vi "Rotate Points.vi"(0 "Points In":cluster{i32, i32}[](array[cluster]), 5 "direction":cluster{"x":i16, "y":i16}, 11 "angle":dbl) -> (4 "Rotated Points":cluster{i32, i32}[](array[cluster]))   [LabVIEW 2020, in "FSM.EdgeEnd.lvclass"]
uses:
  FSM.EdgeEnd.lvclass
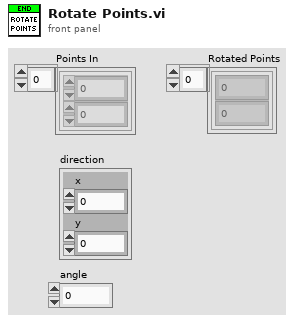
[diagram p1: front panel]
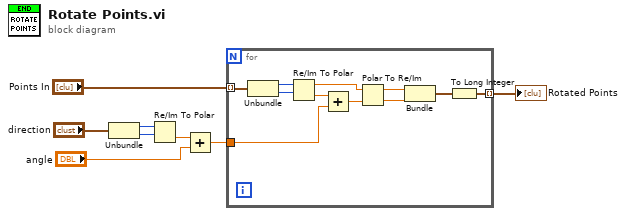
[diagram p0: block diagram]
diagram:
  n1 = Unbundle("direction") -> ("x"=w7:i16, "y"=w6:i16)
  n2 = Re/Im To Polar(2:w6, 3:w7) -> (0:w4:dbl)  [unwired: 1 out]
  n3 = Add(x=w4, y="angle") -> (x+y=w2:dbl)
  n4 = for {
    tunnel: "Points In" -> [w17] mode=indexing
    tunnel: w2 -> [w15]
    tunnel: [w9] -> w3 mode=indexing
    n5 = Unbundle(w17) -> (w19:i32, w18:i32)
    n6 = Re/Im To Polar(2:w18, 3:w19) -> (0:w16:dbl, 1:w13:dbl)
    n7 = Add(x=w16, y=w15) -> (x+y=w14:dbl)
    n8 = Polar To Re/Im(2:w14, 3:w13) -> (0:w11:dbl, 1:w12:dbl)
    n9 = Bundle(w12, w11) -> (w10:cluster{dbl, dbl})  [unwired: 1 in]
    n10 = To Long Integer(number=w10) -> (32bit integer=w9:cluster{i32, i32})
  }
  "Rotated Points" <- w3
